vi "SetIFGateTrackPropPos.vi"(8 "错误输入（无错误）":errorcluster, 10 "闸门跟踪属性":u16) -> (0 "错误输出":errorcluster)   [LabVIEW 2014]
uses:
  ZXUTConfigMgr.dll
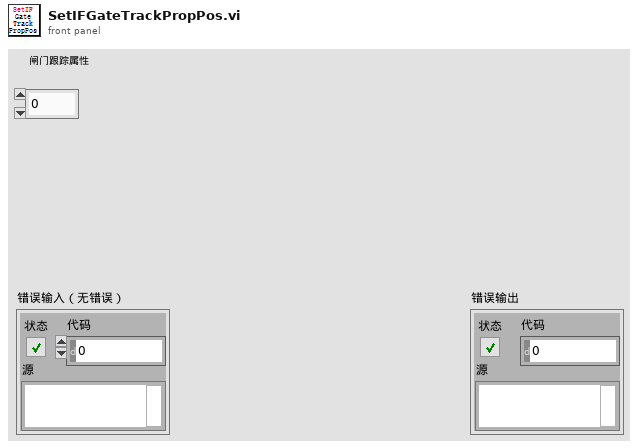
[diagram p1: front panel]
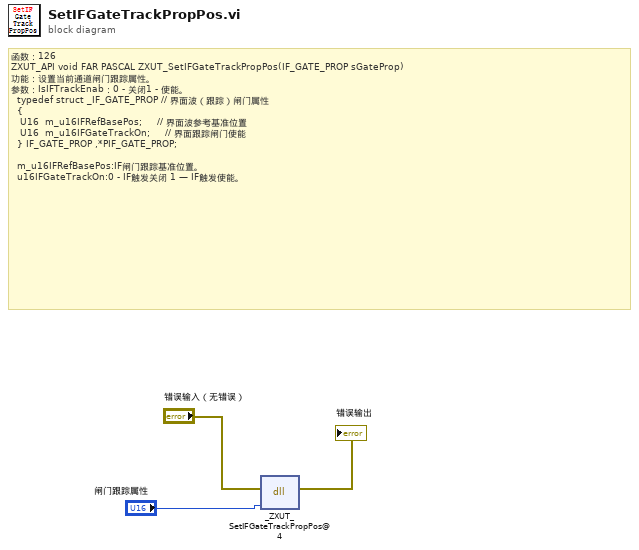
[diagram p0: block diagram]
diagram:
  # "函数：126\nZXUT_API void FAR PASCAL ZXUT_SetIFGateTrackPropPos(IF_GATE_PROP sGateProp)\n功能：设置当前通道闸门跟踪属性。\n参数：IsIFTrackEnab：0 - 关闭1 - 使能。\n\t\ttypedef struct _IF_GATE_PROP\t// 界面波（跟踪）闸门属性\n\t\t{\n\t\t\tU16\t\tm_u16IFRefBasePos;\t\t\t\t\t// 界面波参考基准位置\n\t\t\tU16\t\tm_u16IFGateTrackOn;\t\t\t\t\t// 界面跟踪闸门使能\n\t\t} IF_GATE_PROP ,*PIF_GATE_PROP;\n\n\t\tm_u16IFRefBasePos:IF闸门跟踪基准位置。\n\t\tu16IFGateTrackOn:0 - IF触发关闭 1 — IF触发使能。"
  n1 = dll-call lib="PTH2eabs D软件超声实时监测软件ZXUTAppDemo(华南理工V02.00)X86DllZXUTConfigMgr.dll" fn="_ZXUT_SetIFGateTrackPropPos@4"(error in="错误输入（无错误）", "IsIFTrackEnab"="闸门跟踪属性") -> (error out=→"错误输出":errorcluster)  [unwired: 4 in, 1 out]
